vi "myRIO_BRig_RT__Case_Exp_State_ENL1.vi"(6 "input_LC":bool, 7 "I_lick":bool, 8 "input_LC_led":bool, 10 "input_state":T1, 11 "input_dataCurrent":u16[](array[numeric])) -> (0 "output_trigger_laser_led":bool, 2 "output_state":T1, 3 "output_dataCurrent":u16[](array[numeric]), 4 "output_trigger_laser":bool)   [LabVIEW 2014]
uses:
  myRIO_BRig_RT__Case_Exp_stateList.ctl
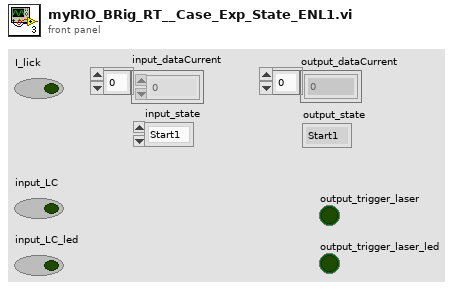
[diagram p1: front panel]
types:
  T1 = typedef "myRIO_BRig_RT__Case_Exp_stateList.ctl" = enum16{"Start1", "Start2", "Start3", "saveSettings1", "saveSettings2", "saveSettings3", "saveSettings4_LC_ENL", "saveSettings5_LC_Cue", "saveSettings6_LC_Other", "setSettings_Audio", "setSettings_Laser", "initBlock_pre", "initBlock", "initBlock2", "initBlock_post", "initTrial_pre", "initTrial", "initTrial2", "initTrial3", "initTrial4", "initTrial_LC_ENL1", "initTrial_LC_Cue1", "initTrial_LC_Sel", "initTrial_post", "ENL1_pre", "ENL1", "ENL1_post", "ENL1Penalty_pre", "ENL1Penalty", "ENL2_pre", "ENL2", "ENL2Penalty_pre", "ENL2Penalty", "Cue1_pre", "Cue1", "Cue1_post", "Cue1Penalty_pre", "Cue1Penalty", "Cue2_pre", "Cue2", "Cue2Penalty_pre", "Cue2Penalty", "Selection_pre", "Selection", "Select_post", "SelectReward_pre", "SelectReward", "SelectRewardPost_pre", "SelectRewardPost", "SelectWrong_pre", "SelectWrong", "SelectWrong_post", "SelectTimeout_pre", "SelectTimeout", "SelectTimeout_post", "endTrial_pre", "endTrial1", "endTrial2", "endTrial3", "endTrial_post", "endBlock_pre", "endBlock", "endBlock_post", "endExp", "commConnect", "commUpload_pre", "commUpload_dataBlock", "commUpload_dataCurrent", "commUpload_dataExp", "commUpload_dataLC", "commUpload_dataTrial", "commUpload_post", "saveData_pre", "saveData_dataBlock", "saveData_dataCurrent", "saveData_dataExp", "saveData_dataLC", "saveData_dataTrial", "saveData_post", "empty_endBlock1", "empty_endBlock2", "empty_endTrial1", "empty_endTrial2", "empty_endTrial3", "empty_endTrial4", "empty_endTrial5", "dummyState", "dummyState_endBlock"}
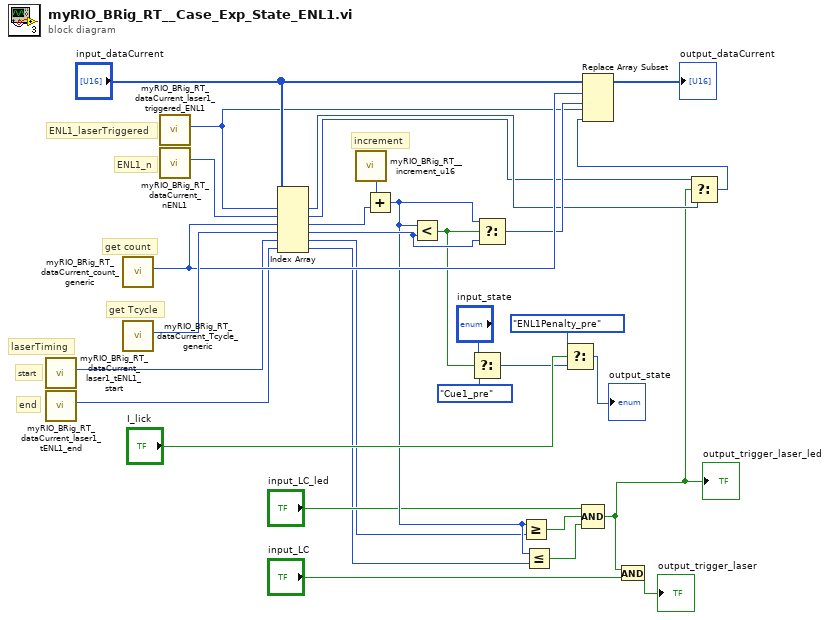
[diagram p0: block diagram]
diagram:
  # "ENL1_laserTriggered"
  # "ENL1_n"
  # "end"
  # "start"
  # "laserTiming"
  # "increment"
  # "get Tcycle"
  # "get count"
  n1 = call "myRIO_BRig_RT_dataCurrent_laser1_tENL1_start.vi"() -> ("output_laser1_tENL1_start"=w11:i32)  [unwired: 11 in]
  n2 = call "myRIO_BRig_RT_dataCurrent_laser1_tENL1_end.vi"() -> ("output_laser1_tENL1_end"=w10:i32)  [unwired: 11 in]
  n3 = call "myRIO_BRig_RT_dataCurrent_count_generic.vi"() -> ("output_count_generic"=w27:i32)  [unwired: 11 in]
  n4 = call "myRIO_BRig_RT_dataCurrent_Tcycle_generic.vi"() -> ("output_Tcycle_generic"=w29:i32)  [unwired: 11 in]
  n5 = call "myRIO_BRig_RT_dataCurrent_laser1_triggered_ENL1.vi"() -> ("output_laser1_triggered_ENL1"=w6:i32)  [unwired: 11 in]
  n6 = call "myRIO_BRig_RT_dataCurrent_nENL1.vi"() -> ("output_nENL1"=w7:i32)  [unwired: 11 in]
  n7 = Index Array(array="input_dataCurrent", index #1=w6, index #2=w7, index #3=w27, index #4=w29, index #5=w11, index #6=w10) -> (element #1=w5:u16, element #2=w4:u16, element #3=w28:u16, element #4=w26:u16, element #5=w9:u16, element #6=w8:u16)
  n8 = call "myRIO_BRig_RT__increment_u16.vi"() -> ("output_increment__u16"=w20:u16)  [unwired: 11 in]
  n9 = Add(x=w20, y=w28) -> (x+y=w19:u16)
  n10 = Less?(x=w19, y=w26) -> (x < y?=w23:bool)
  n11 = Select(t="input_state", s=w23, f=myRIO_BRig_RT__Case_Exp_stateList."Cue1_pre" ("Enum")) -> (s? t:f=w22:T1)
  n12 = Select(t=w19, s=w23, f=w26) -> (s? t:f=w25:u16)
  n13 = Greater Or Equal?(x=w19, y=w9) -> (x >= y?=w17:bool)
  n14 = Less Or Equal?(x=w19, y=w8) -> (x <= y?=w18:bool)
  n15 = Select(t=myRIO_BRig_RT__Case_Exp_stateList."ENL1Penalty_pre" ("Enum"), s="I_lick", f=w22) -> (s? t:f=→"output_state":T1)
  n16 = Compound Arithmetic op=AND("input_LC_led", w17, w18) -> (w2:bool)
  "output_trigger_laser_led" <- w2
  n17 = And(x=w2, y="input_LC") -> (x .and. y?=→"output_trigger_laser":bool)
  n18 = Select(t=w4, s=w2, f=w5) -> (s? t:f=w3:u16)
  n19 = Replace Array Subset(array="input_dataCurrent", new element #1=w25, index #1=w27, new element #2=w3, index #2=w6) -> (→"output_dataCurrent":u16[])
